vi "All Unit Tests.vi"() -> ()   [LabVIEW 2019, in "Sports Unit Tests.lvclass"]
uses:
  Sports Unit Tests.lvclass
  <vilib>/addons/_JKI Toolkits/Caraya/run-tests/Run Test (Object).vi
  <vilib>/addons/_JKI Toolkits/Caraya/Caraya.lvlib
panel:
  out "error out":errorcluster
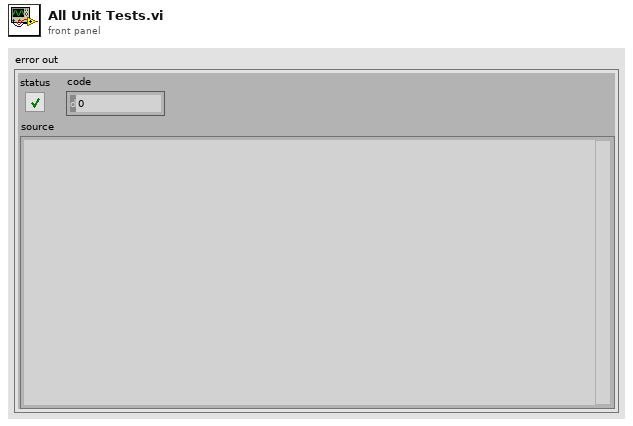
[diagram p1: front panel]
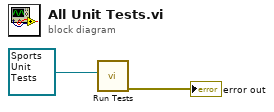
[diagram p0: block diagram]
diagram:
  n1 = call-poly <vilib>:"Run Tests.vi"("Object"=refnum<class "Sports Unit Tests.lvclass"> refnum ("Sports Unit Tests.lvclass")) -> ("error out"=→"error out":errorcluster)  [unwired: 10 in]
